vi "TestSaveAPDInfo.vi"() -> ()   [LabVIEW 2020]
uses:
  SubVI/APD/APDClass.lvclass
panel:
  in  "error in (no error)":errorcluster
  out "Error Out":errorcluster
  out "Gain":cluster{"v":dbl[], "y":dbl[]}(graph)
  out "iRF":cluster{"x":i32[], "y":dbl[]}(graph)
  in  "APD Serial #":string="M00549706"
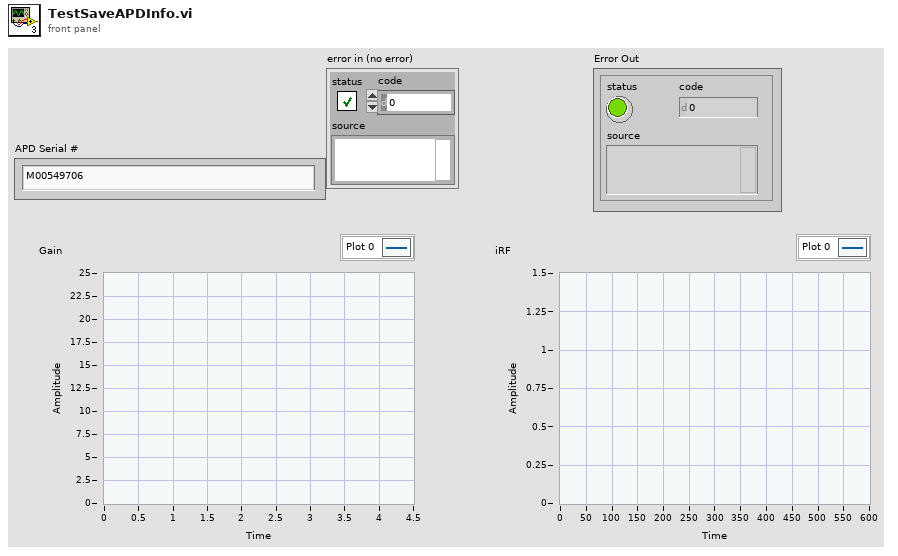
[diagram p1: front panel]
types:
  T1 = cluster{"CtrlV":dbl[], "Gain":dbl[], "GainRaw":dbl[][]}
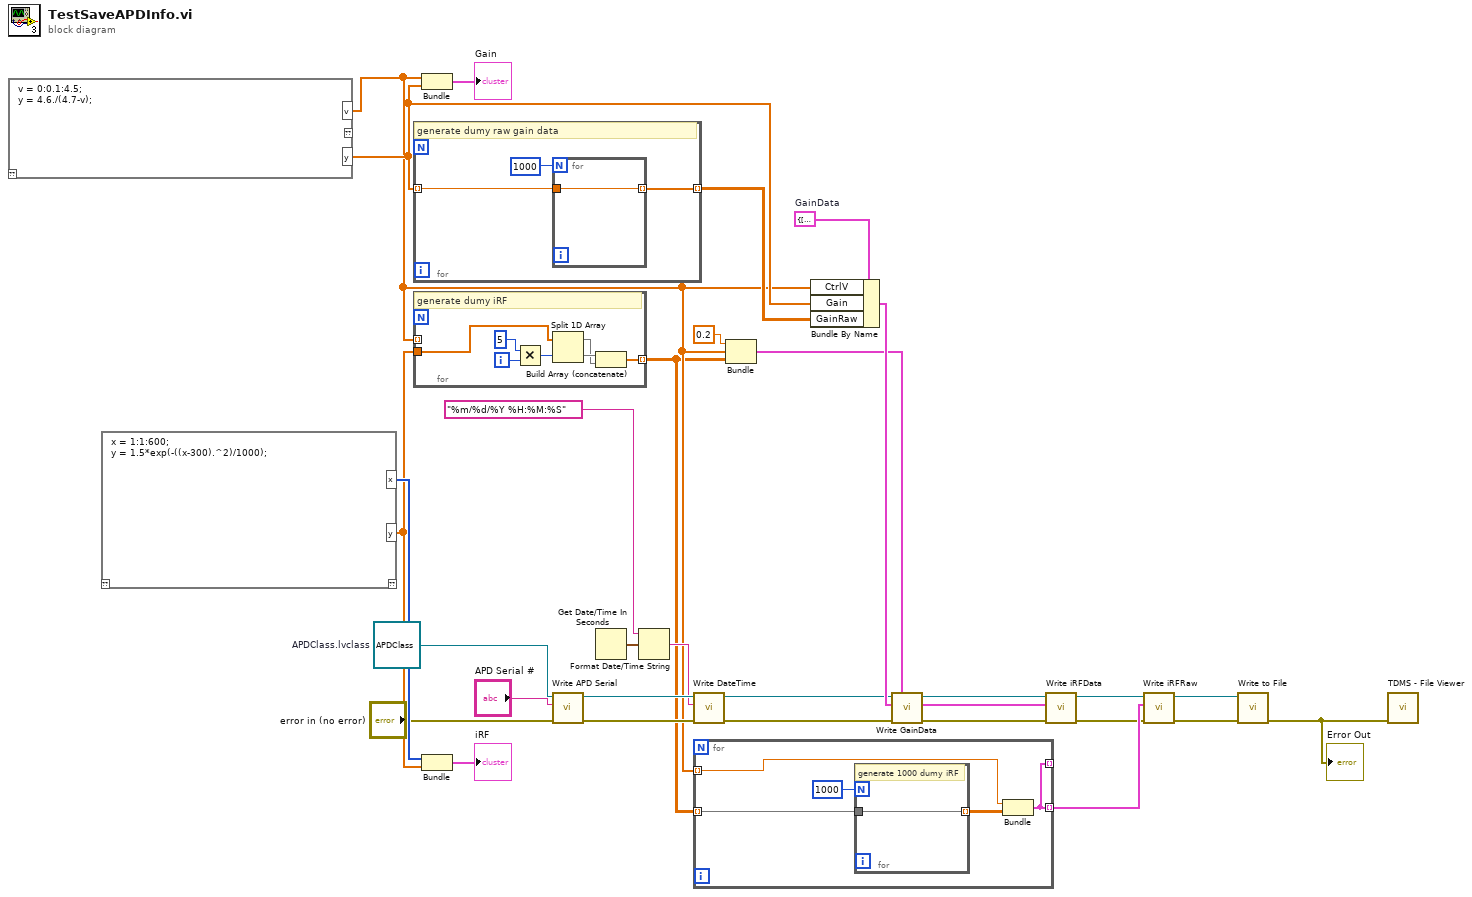
[diagram p0: block diagram]
diagram:
  w1 = T1 {"CtrlV"=[], "Gain"=[], "GainRaw"=[]}  # GainData
  w19 = refnum<class "APDClass.lvclass"> refnum  # APDClass.lvclass
  n1 = mathscript code="v = 0:0.1:4.5;\ny = 4.6./(4.7-v);"() -> ("y"=w25:dbl[], "v"=w10:dbl[])  [unwired: 1 in, 1 out]
  n2 = mathscript code="x = 1:1:600;\ny = 1.5*exp(-((x-300).^2)/1000);"() -> ("y"=w27:dbl[], "x"=w30:i32[])  [unwired: 1 in, 1 out]
  n3 = for {
    tunnel: w25 -> [w32] mode=indexing
    tunnel: [w31] -> w24 mode=indexing
    # "generate dumy raw gain data"
    n4 = for {
      N: 1000 -> [_]
      tunnel: w32 -> [w34]
      tunnel: [w34] -> w31 mode=indexing
    }
  }
  n5 = for {
    tunnel: w10 -> [_] mode=indexing
    tunnel: w27 -> [w41]
    tunnel: [w35] -> w9 mode=indexing
    i -> [w40]
    # "generate dumy iRF"
    n6 = Multiply(x=5, y=w40) -> (x*y=w38:i32)
    n7 = Split 1D Array(array=w41, index=w38) -> (first subarray=w36:dbl[], second subarray=w37:dbl[])
    n8 = Build Array (concatenate)(w37, w36) -> (w35:dbl[])
  }
  n9 = Bundle("v"=w10, "y"=w25) -> (→"Gain":cluster{"v":dbl[], "y":dbl[]})  [unwired: 1 in]
  n10 = Bundle("x"=w30, "y"=w27) -> (→"iRF":cluster{"x":i32[], "y":dbl[]})  [unwired: 1 in]
  n11 = call-dynamic "Write APD Serial.vi"("error in (no error)"="error in (no error)", "APD Serial #"="APD Serial #", "APDClass in"=w19) -> ("error out"=w15:errorcluster, "APDClass out"=w17:refnum<class "APDClass.lvclass">)  [unwired: 7 in]
  n12 = Get Date/Time In Seconds() -> (seconds since 1Jan1904=w13:timestamp)
  n13 = Format Date/Time String(time format string (%c)="%m/%d/%Y %H:%M:%S", seconds (now)=w13) -> (date/time string=w11:string)  [unwired: 1 in]
  n14 = call-dynamic "Write DateTime.vi"("error in (no error)"=w15, "DateTime"=w11, "APDClass in"=w17) -> ("error out"=w14:errorcluster, "APDClass out"=w16:refnum<class "APDClass.lvclass">)  [unwired: 7 in]
  n15 = for {
    tunnel: w10 -> [w46] mode=indexing
    tunnel: w9 -> [w45] mode=indexing
    tunnel: [w42] -> _ mode=indexing
    tunnel: [w42] -> w8 mode=indexing
    n16 = for {
      N: 1000 -> [_]
      tunnel: w45 -> [w47]
      tunnel: [w47] -> w43 mode=indexing
      # "generate 1000 dumy iRF"
    }
    n17 = Bundle(w46, w43) -> (w42:cluster{dbl, dbl[][]})  [unwired: 1 in]
  }
  n18 = Bundle(0.2, "v"=w10, w9) -> (w22:cluster{dbl, "v":dbl[], dbl[][]})  [unwired: 1 in]
  n19 = Bundle By Name(cluster=w1, "CtrlV"=w10, "Gain"=w25, "GainRaw"=w24) -> (w23:T1)
  n20 = call-dynamic "Write GainData.vi"("error in (no error)"=w14, "GainData"=w23, "APDClass in"=w16) -> ("error out"=w20:errorcluster, "APDClass out"=w21:refnum<class "APDClass.lvclass">)  [unwired: 7 in]
  n21 = call-dynamic "Write iRFData.vi"("error in (no error)"=w20, "iRFData"=w22, "APDClass in"=w21) -> ("error out"=w6:errorcluster, "APDClass out"=w7:refnum<class "APDClass.lvclass">)  [unwired: 7 in]
  n22 = call-dynamic "Write iRFRaw.vi"("error in (no error)"=w6, "iRFRaw"=w8, "APDClass in"=w7) -> ("error out"=w4:errorcluster, "APDClass out"=w5:refnum<class "APDClass.lvclass">)  [unwired: 7 in]
  n23 = call "Write to File.vi"("Error In"=w4, "APDClass.lvclass"=w5) -> ("Error Out"=w2:errorcluster)  [unwired: 9 in]
  "Error Out" <- w2
  n24 = call <vilib>:"TDMS - File Viewer.vi"("error in (no error)"=w2) -> ()  [unwired: 5 in, 2 out]
